vi "SetProgramParameters.vi"(8 "error in (no error)":errorcluster, 9 "Port Type":enum16{"GPIB", "Serial"}(ring), 10 "Handle":string, 11 "Waveform":T1) -> (0 "error out":errorcluster)   [LabVIEW 2018, in "AcPwrPlugins.lvlib" / "PacificPowerSource.lvclass"]
uses:
  PacificPowerSource.lvclass
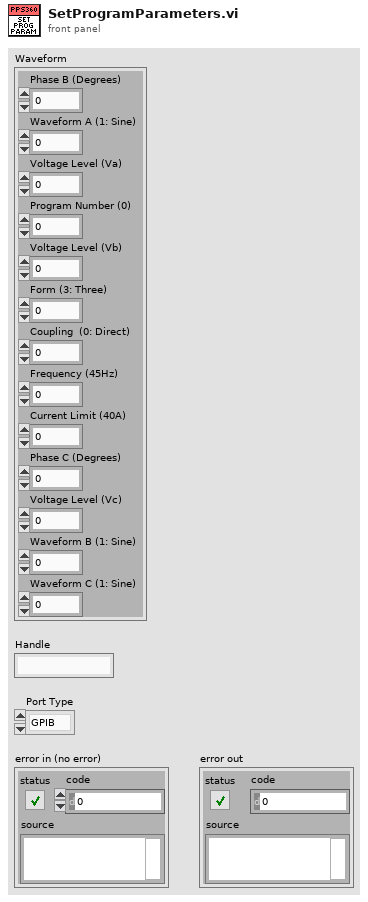
[diagram p1: front panel]
types:
  T1 = cluster{"Phase B (Degrees)":i32, "Waveform A (1: Sine)":i32, "Voltage Level (Va)":dbl, "Program Number (0)":i32, "Voltage Level (Vb) ":dbl, "Form (3: Three)":u16, "Coupling  (0: Direct)":u16, "Frequency (45Hz)":dbl, "Current Limit (40A)":dbl, "Phase C (Degrees)":i32, "Voltage Level (Vc)":dbl, "Waveform B (1: Sine)":i32, "Waveform C (1: Sine)":i32}
  T2 = cluster{"Waveform 1":i32, "Waveform 2":i32, "Waveform 3":i32, "Voltage 1":dbl, "Voltage 2":dbl, "Voltage 3":dbl, "Phase 2":dbl, "Phase 3":dbl, "Frequency":dbl, "Current Limit":dbl, "# of Trans Events":i32, "Form":u16, "Coupling":u16, "XFMR Ratio":dbl, "Exec Angle":dbl}
  T3 = cluster{"Program Name":i32, "Waveform 1":i32, "Waveform 2":i32, "Waveform 3":i32, "Voltage 1":dbl, "Voltage 2":dbl, "Voltage 3":dbl, "Phase 2":dbl, "Phase 3":dbl, "Frequency":dbl, "Current Limit":dbl, "No. of Trans Events":i32, "Form":u16, "Coupling":u16, "XFMR Ratio":dbl, "Exec Angle":dbl}
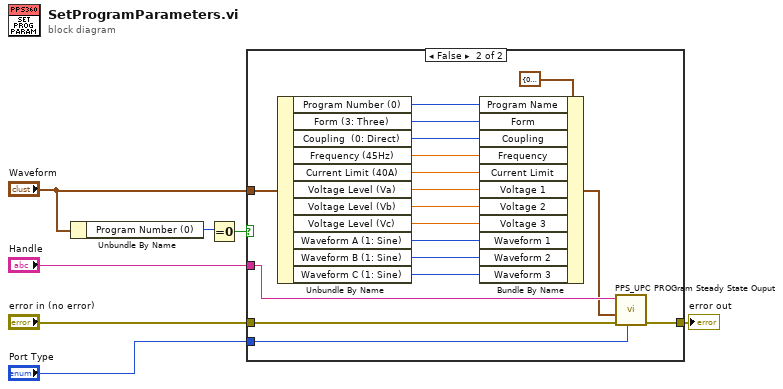
[diagram p0: block diagram]
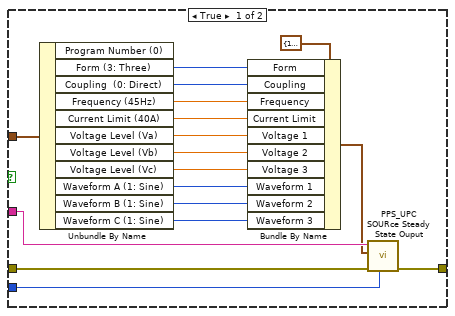
[diagram p2: hidden frame]
diagram:
  n1 = Unbundle By Name("Waveform") -> ("Program Number (0)"=w3:i32)
  n2 = Equal To 0?(x=w3) -> (x = 0?=w4:bool)
  n3 = case shown="False" w4 {
    tunnel: "error in (no error)" -> [w24 w42]
    tunnel: [w23 w31] -> w2
    tunnel: "Port Type" -> [w22 w30]
    tunnel: "Handle" -> [w21 w29]
    tunnel: "Waveform" -> [w19 w41]
    frame True {
      n4 = Unbundle By Name(w19) -> ("Form (3: Three)"=w9:u16, "Coupling  (0: Direct)"=w10:u16, "Frequency (45Hz)"=w14:dbl, "Current Limit (40A)"=w15:dbl, "Voltage Level (Va)"=w18:dbl, "Voltage Level (Vb)"=w17:dbl, "Voltage Level (Vc)"=w16:dbl, "Waveform A (1: Sine)"=w13:i32, "Waveform B (1: Sine)"=w12:i32, "Waveform C (1: Sine)"=w11:i32)  [unwired: 1 out]
      n5 = Bundle By Name(cluster=T2 {"Waveform 1"=1, "Waveform 2"=1, "Waveform 3"=1, "Voltage 1"=100.0, "Voltage 2"=100.0, "Voltage 3"=100.0, "Phase 2"=120.0, "Phase 3"=240.0, "Frequency"=100.0, "Current Limit"=10.0, "# of Trans Events"=0, "Form"=0, "Coupling"=0, "XFMR Ratio"=0.0, "Exec Angle"=0.0} ("Steady State Output Parameters 2"), "Form"=w9, "Coupling"=w10, "Frequency"=w14, "Current Limit"=w15, "Voltage 1"=w18, "Voltage 2"=w17, "Voltage 3"=w16, "Waveform 1"=w13, "Waveform 2"=w12, "Waveform 3"=w11) -> (w20:T2)
      n6 = call <instrlib>:"PPS_UPC SOURce Steady State Ouput.vi"("Port Type"=w22, "error in (no error)"=w24, "Steady State\nOutput Parameters"=w20, "VISA session"=w21) -> ("error out"=w23:errorcluster)  [unwired: 6 in, 1 out]
    }
    frame False {
      n7 = Unbundle By Name(w41) -> ("Program Number (0)"=w27:i32, "Form (3: Three)"=w28:u16, "Coupling  (0: Direct)"=w32:u16, "Frequency (45Hz)"=w36:dbl, "Current Limit (40A)"=w37:dbl, "Voltage Level (Va)"=w40:dbl, "Voltage Level (Vb)"=w39:dbl, "Voltage Level (Vc)"=w38:dbl, "Waveform A (1: Sine)"=w35:i32, "Waveform B (1: Sine)"=w34:i32, "Waveform C (1: Sine)"=w33:i32)
      n8 = Bundle By Name(cluster=T3 {"Program Name"=0, "Waveform 1"=0, "Waveform 2"=0, "Waveform 3"=0, "Voltage 1"=0.0, "Voltage 2"=0.0, "Voltage 3"=0.0, "Phase 2"=0.0, "Phase 3"=0.0, "Frequency"=0.0, "Current Limit"=0.0, "No. of Trans Events"=0, "Form"=0, "Coupling"=0, "XFMR Ratio"=0.0, "Exec Angle"=0.0} ("Program Steady State Parameters"), "Program Name"=w27, "Form"=w28, "Coupling"=w32, "Frequency"=w36, "Current Limit"=w37, "Voltage 1"=w40, "Voltage 2"=w39, "Voltage 3"=w38, "Waveform 1"=w35, "Waveform 2"=w34, "Waveform 3"=w33) -> (w26:T3)
      n9 = call <instrlib>:"PPS_UPC PROGram Steady State Ouput.vi"("Port Type"=w30, "error in (no error)"=w42, "Program Steady State Parameters"=w26, "VISA session"=w29) -> ("error out"=w31:errorcluster)  [unwired: 6 in, 1 out]
    }
  }
  "error out" <- w2
